vi "Simultaneous Sound IO.vi"() -> ()   [LabVIEW 2014]
doc: "This VI illustrates how to perform simultaneous sound IO, i.e., how to continuously play the sound acquired from a microphone. It requires the use of a microphone attached to the sound card. You can specify the IDs of the input and output devices, the frequency to sample at, and the buffer size for both devices. Higher frequencies have better quality, but demand more resources and are limited by the capabilities of your sound card. A large number of samples decreases the risk of glitches, but increases the delay between acquisition and playback."
uses:
  <vilib>/sound2/lvsound2.llb/Sound Data Format.ctl
  <vilib>/sound2/lvsound2.llb/Sampling Mode.ctl
  <vilib>/sound2/lvsound2.llb/Sound Output Write (DBL Single).vi
  <vilib>/sound2/lvsound2.llb/Sound Input Read (DBL).vi
  <vilib>/sound2/lvsound2.llb/Sound Output Write (DBL).vi
panel:
  out "Filtered Data":waveform(dbl)[](graph)
  out "Raw Data":waveform(dbl)[](graph)
  in  "Sound Format":T1={"sample rate (S/s)"=44100.0, "number of channels"=2, "bits per sample"=16}
  in  "stop":bool
  in  "Number of Samples/ch":i32=20000
  in  "Input Device ID":u32
  in  "Output Device ID":u32
  # "This VI continuously plays the sound acquired from a microphone.\n\nInstructions to execute the VI:\n1.  Specify the IDs of the input and output devices, the frequency to sample at, and the buffer size for both devices. Higher frequencies have better quality, but demand more resources and are limited by the capabilities of your sound card.  A large number of samples decreases the risk of glitches, but increases the delay between acquisition and playback.\n2.  Run the VI.\n3.  Press the Stop button when done."
  # "Configuration"
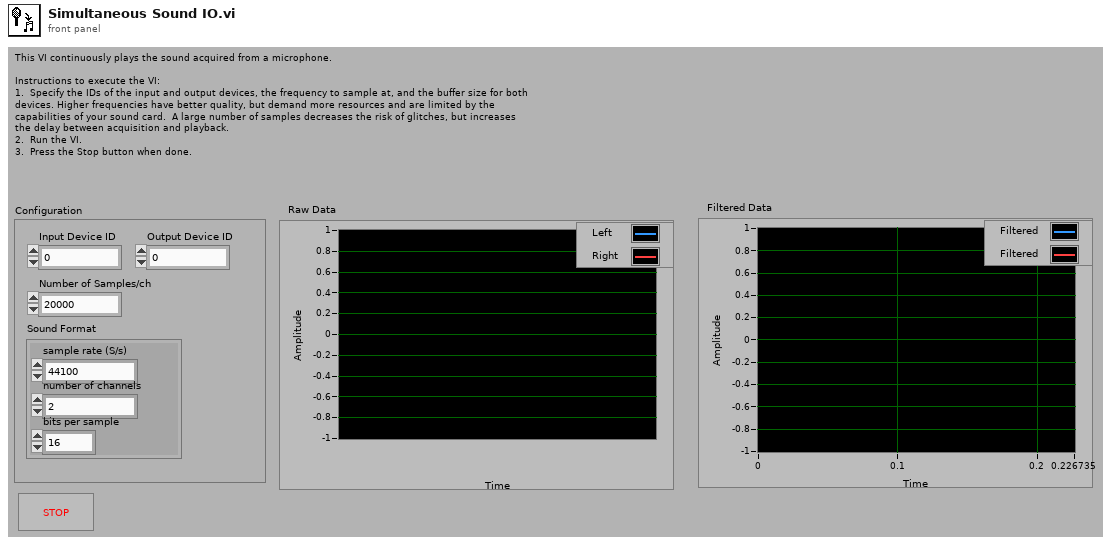
[diagram p1: front panel]
types:
  T1 = typedef "Sound Data Format.ctl" = cluster{"sample rate (S/s)":dbl, "number of channels":i32, "bits per sample":i32}
  T2 = typedef "Sampling Mode.ctl" = i32
  T3 = typedef "Sound Output Task ID.ctl" = u32
  T4 = typedef "Sound Input Task ID.ctl" = u32
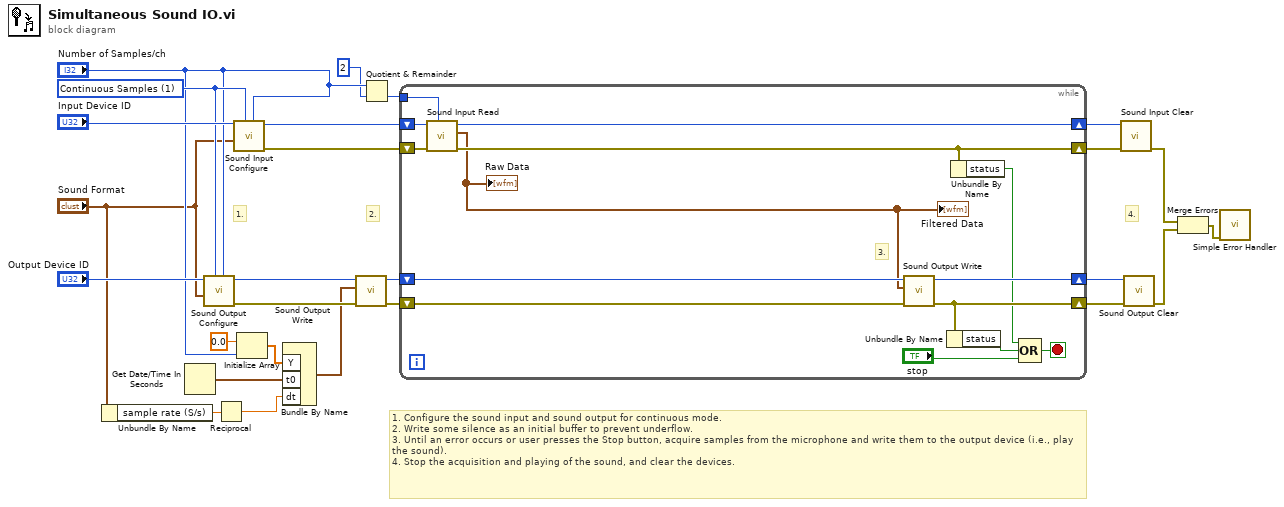
[diagram p0: block diagram]
diagram:
  w16 = T2 1 items=["Finite Samples", "Continuous Samples"] ("sample mode")
  # "2."
  # "4."
  # "1."
  # "1. Configure the sound input and sound output for continuous mode.\n2. Write some silence as an initial buffer to prevent underflow.\n3. Until an error occurs or user presses the Stop button, acquire samples from the microphone and write them to the output device (i.e., play the sound).\n4. Stop the acquisition and playing of the sound, and clear the devices."
  n1 = Unbundle By Name("Sound Format") -> ("sample rate (S/s)"=w3:dbl)
  n2 = Get Date/Time In Seconds() -> (seconds since 1Jan1904=w1:timestamp)
  n3 = call <vilib>:"Sound Output Configure.vi"("number of samples/ch"="Number of Samples/ch", "sample mode"=w16, "sound format"="Sound Format", "device ID"="Output Device ID") -> ("error out"=w14:errorcluster, "task ID"=w15:T3)  [unwired: 6 in]
  n4 = Reciprocal(x=w3) -> (1/x=w2:dbl)
  n5 = call <vilib>:"Sound Input Configure.vi"("number of samples/ch"="Number of Samples/ch", "sample mode"=w16, "sound format"="Sound Format", "device ID"="Input Device ID") -> ("error out"=w18:errorcluster, "task ID"=w17:T4)  [unwired: 6 in]
  n6 = Initialize Array(0.0 ("element"), "Number of Samples/ch") -> (w5:dbl[])
  n7 = Bundle By Name("Y"=w5, "t0"=w1, "dt"=w2) -> (w6:waveform(dbl))  [unwired: 1 in]
  n8 = call-poly <vilib>:"Sound Output Write.vi"("error in (no error)"=w14, "data"=w6, "task ID"=w15) -> ("error out"=w13:errorcluster, "task ID out"=w12:T3)  [unwired: 7 in]
  n9 = Quotient & Remainder(x="Number of Samples/ch", y=2) -> (floor(x/y)=w9:i32)  [unwired: 1 out]
  n10 = while {
    shift-right: [w32] -> w25
    shift-left: w13 -> [w34]
    shift-right: [w33] -> w26
    shift-left: w18 -> [w40]
    tunnel: w9 -> [w36]
    shift-right: [w37] -> w24
    shift-left: w12 -> [w39]
    shift-right: [w35] -> w21
    shift-left: w17 -> [w38]
    stop <- w28 stop-if-true
    # "3."
    n11 = call-poly <vilib>:"Sound Input Read.vi"("number of samples/ch"=w36, "error in (no error)"=w40, "task ID"=w38) -> ("error out"=w33:errorcluster, "data"=w27:waveform(dbl)[], "task ID out"=w35:T4)  [unwired: 6 in]
    "Raw Data" <- w27
    "Filtered Data" <- w27
    n12 = call-poly <vilib>:"Sound Output Write.vi"("error in (no error)"=w34, "data"=w27, "task ID"=w39) -> ("error out"=w32:errorcluster, "task ID out"=w37:T3)  [unwired: 7 in]
    n13 = Unbundle By Name(w32) -> ("status"=w30:bool)
    n14 = Unbundle By Name(w33) -> ("status"=w29:bool)
    n15 = Compound Arithmetic op=OR(w29, w30, "stop") -> (w28:bool)
  }
  n16 = call <vilib>:"Sound Input Clear.vi"("error in (no error)"=w26, "task ID"=w21) -> ("error out"=w19:errorcluster)  [unwired: 9 in]
  n17 = call <vilib>:"Sound Output Clear.vi"("error in (no error)"=w25, "task ID"=w24) -> ("error out"=w20:errorcluster)  [unwired: 9 in]
  n18 = Merge Errors(w19, w20) -> (w11:errorcluster)
  n19 = call <vilib>:"Simple Error Handler.vi"("error in (no error)"=w11) -> ()  [unwired: 4 in, 5 out]
